vi "KepcoDCPwr Query Voltage Protect Unit Limit.vi"(0 "VISA Session":refnum<visa-resource-name>, 5 "Model In":string, 7 "channel name (\"\")":string="\"\"", 9 "Max Level (T),MIN LEVEL(F)":bool caption="Level", 11 "error in (no error)":errorcluster {"code" format="%.0x"}) -> (4 "VISA Session Out":refnum<visa-resource-name>, 6 "Model Out":string, 8 "channel name out (\"\")":string="\"\"" caption="channel name Out (\"\")", 10 "voltage level":dbl format="%^.2e", 15 "error out":errorcluster {"code" format="%.0x"})   [LabVIEW 2010]
doc: "This VI returns the maximum programmable voltage protect level that the power supply accepts. This limit may be configurable to find out unit limits use Volt Protect unit limit"
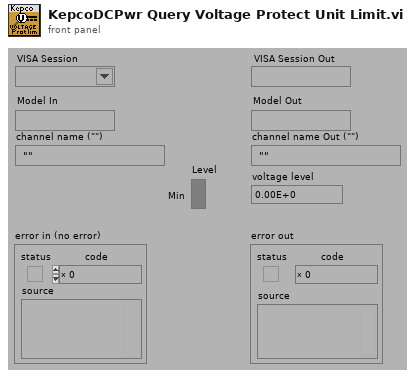
[diagram p1: front panel]
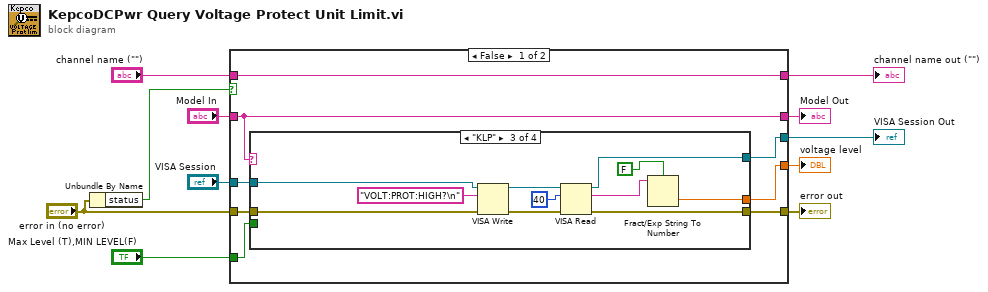
[diagram p0: block diagram]
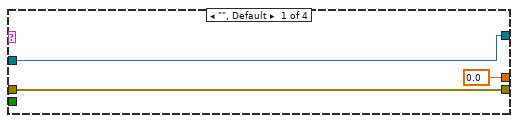
[diagram p2: hidden frame]
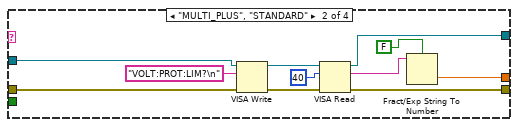
[diagram p3: hidden frame]
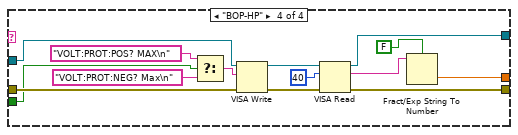
[diagram p4: hidden frame]
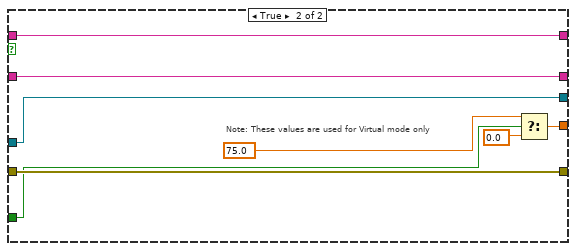
[diagram p5: hidden frame]
diagram:
  n1 = Unbundle By Name("error in (no error)") -> ("status"=w10:bool)
  n2 = case shown="False" w10 {
    tunnel: [w14 w66] -> w11
    tunnel: "error in (no error)" -> [w17 w66]
    tunnel: [w15 w65] -> w5
    tunnel: "VISA Session" -> [w18 w65]
    tunnel: [w16 w64] -> w4
    tunnel: "Model In" -> [w16 w64]
    tunnel: [w19 w63] -> w3
    tunnel: "channel name (\"\")" -> [w19 w63]
    tunnel: [w13 w60] -> w2
    tunnel: "Max Level (T),MIN LEVEL(F)" -> [w12 w62]
    frame False {
      n3 = case shown="\"KLP\"" w16 {
        tunnel: w17 -> [w22 w33 w44 w58]
        tunnel: w18 -> [w20 w32 w43 w57]
        tunnel: [w20 w30 w41 w56] -> w15
        tunnel: [w22 w29 w40 w55] -> w14
        tunnel: [0.0 w26 w37 w53] -> w13
        tunnel: w12 -> [_ _ _ w51]
        frame "", Default {
        }
        frame "MULTI_PLUS", "STANDARD" {
          n4 = VISA Write(VISA resource name=w32, write buffer="VOLT:PROT:LIM?\n", error in (no error)=w33) -> (VISA resource name out=w31:refnum<visa-resource-name>, error out=w28:errorcluster)  [unwired: 1 out]
          n5 = VISA Read(VISA resource name=w31, byte count=u32 40 ("byte count (0)"), error in (no error)=w28) -> (VISA resource name out=w30:refnum<visa-resource-name>, read buffer=w27:string, error out=w29:errorcluster)  [unwired: 1 out]
          n6 = Fract/Exp String To Number(use system decimal point (T)=FALSE, string=w27) -> (number=w26:dbl)  [unwired: 2 in, 1 out]
        }
        frame "KLP" {
          n7 = VISA Write(VISA resource name=w43, write buffer="VOLT:PROT:HIGH?\n", error in (no error)=w44) -> (VISA resource name out=w42:refnum<visa-resource-name>, error out=w39:errorcluster)  [unwired: 1 out]
          n8 = VISA Read(VISA resource name=w42, byte count=u32 40 ("byte count (0)"), error in (no error)=w39) -> (VISA resource name out=w41:refnum<visa-resource-name>, read buffer=w38:string, error out=w40:errorcluster)  [unwired: 1 out]
          n9 = Fract/Exp String To Number(use system decimal point (T)=FALSE, string=w38) -> (number=w37:dbl)  [unwired: 2 in, 1 out]
        }
        frame "BOP-HP" {
          n10 = Select(t="VOLT:PROT:POS? MAX\n", s=w51, f="VOLT:PROT:NEG? Max\n") -> (s? t:f=w48:string)
          n11 = VISA Write(VISA resource name=w57, write buffer=w48, error in (no error)=w58) -> (VISA resource name out=w46:refnum<visa-resource-name>, error out=w47:errorcluster)  [unwired: 1 out]
          n12 = VISA Read(VISA resource name=w46, byte count=u32 40 ("byte count (0)"), error in (no error)=w47) -> (VISA resource name out=w56:refnum<visa-resource-name>, read buffer=w54:string, error out=w55:errorcluster)  [unwired: 1 out]
          n13 = Fract/Exp String To Number(use system decimal point (T)=FALSE, string=w54) -> (number=w53:dbl)  [unwired: 2 in, 1 out]
        }
      }
    }
    frame True {
      # "Note: These values are used for Virtual mode only"
      n14 = Select(t=75.0, s=w62, f=0.0) -> (s? t:f=w60:dbl)
    }
  }
  "error out" <- w11
  "channel name out (\"\")" <- w3
  "Model Out" <- w4
  "VISA Session Out" <- w5
  "voltage level" <- w2
